vi "Move Drive Encoders.vi"() -> ()   [LabVIEW 2014]
uses:
  Begin/Global RefNums.vi
panel:
  in  "Reset Encoders":bool
  out "BR Current Encoder":i32
  out "BL Current Encoder":i32
  out "FR Current Encoder":i32
  out "FL Current Encoder":i32
  in  "BR Drive Motor":bool
  in  "BL Drive Motor":bool
  in  "FR Drive Motor":bool
  in  "FL Drive Motor":bool
  in  "Drive Back?":bool
  in  "BR Rot Motor":bool
  in  "BL Rot Motor":bool
  in  "FR Rot Motor":bool
  in  "FL Rot Motor":bool
  in  "BR Rot Speed":dbl
  in  "BL Rot Speed":dbl
  in  "FR Rot Speed":dbl
  in  "FL Rot Speed":dbl
  in  "?":bool
  in  "BR Target Encoder":i32
  in  "BL Target Encoder":i32
  in  "FR Target Encoder":i32
  in  "FL Target Encoder":i32
  in  "BR Drive Speed":dbl
  in  "BL Drive Speed":dbl
  in  "FR Drive Speed":dbl
  in  "FL Drive Speed":dbl
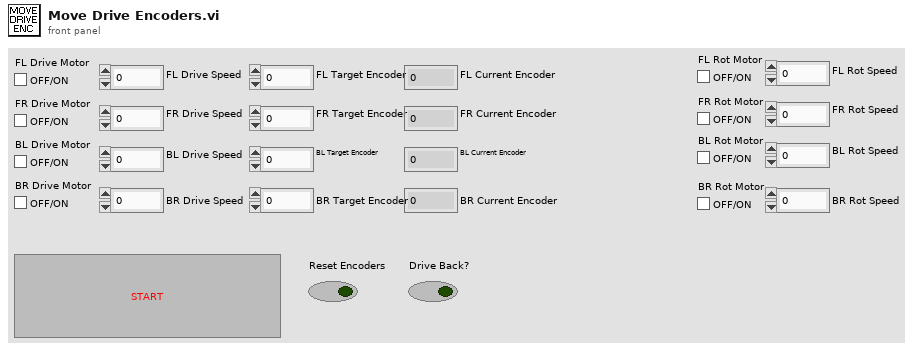
[diagram p1: front panel]
types:
  T1 = typedef "WPI_MotorControlDeviceRef.ctl" = cluster{"DeviceStatus":errorcluster, "Type":T2, "PWM":cluster{"Controller":T3, "PWM Channel":T4, "DeadBand":T5}, "CAN":cluster{"Device Number":u8, "Control Mode":T6, "Semaphore":T7, "Max Vout":dbl, "TalonSRX Control Mode":T8}, "Invert":bool, "TransformRef":T9, "InvTransformRef":T9}
  T2 = typedef "WPI_MotorControlType.ctl" = enum16{"PWM", "CAN", "CANTalonSRX"}
  T3 = typedef "FPGA_TypedefDigitalModule.ctl" = enum16{"Controller 1"}
  T4 = typedef "FPGA_DIOPWMChannel.ctl" = enum8{"PWM 0", "PWM 1", "PWM 2", "PWM 3", "PWM 4", "PWM 5", "PWM 6", "PWM 7", "PWM 8", "PWM 9", "PWM MXP 0", "PWM MXP 1", "PWM MXP 2", "PWM MXP 3", "PWM MXP 4", "PWM MXP 5", "PWM MXP 6", "PWM MXP 7", "PWM MXP 8", "PWM MXP 9", "Invalid"}
  T5 = typedef "WPI_PWMDeadband.ctl" = cluster{"Name":string, "maxPositivePwm":i32, "minPositivePwm":i32, "centerPwm":i32, "maxNegativePwm":i32, "minNegativePwm":i32, "angularRange":u16}
  T6 = typedef "WPI_CANJaguar_ControlMode.ctl" = enum8{"Percent VBus", "Current", "Speed", "Position", "Voltage"}
  T7 = typedef "Semaphore RefNum" = refnum<k1>
  T8 = typedef "WPI_CANTalonSRX_APIControlMode.ctl" = enum8{"Percent VBus", "Speed", "Position", "Slave", "Unchanged / Invalid"}
  T9 = typedef "WPI_PWMTransform_ConPane.ctl" = refnum<vi>
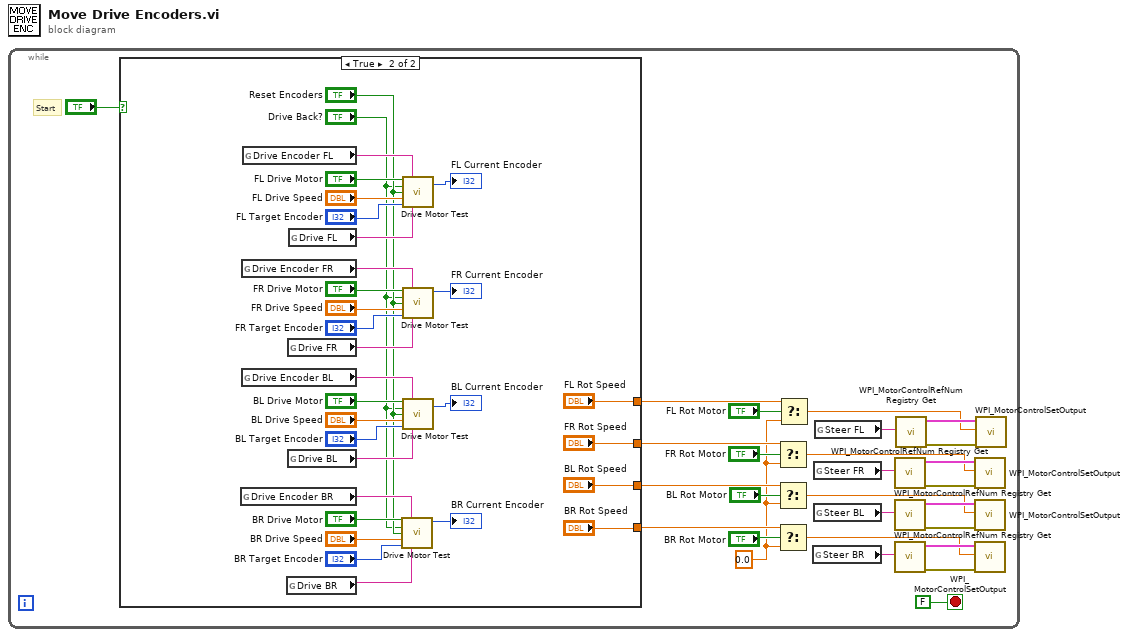
[diagram p0: block diagram]
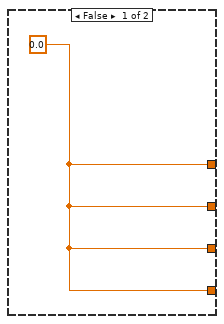
[diagram p2: hidden frame]
diagram:
  n1 = while {
    stop <- FALSE stop-if-true
    w1 = 0.0 ("f")
    # "Start"
    n2 = case shown="True" "?" {
      tunnel: [w28 "FL Rot Speed"] -> w5
      tunnel: [w28 "FR Rot Speed"] -> w4
      tunnel: [w28 "BL Rot Speed"] -> w3
      tunnel: [w28 "BR Rot Speed"] -> w2
      frame False {
        w28 = 0.0 ("FL Drive Speed")
      }
      frame True {
        n3 = global read "Global RefNums.vi" "Drive Encoder BR"() -> (w41:string)
        n4 = global read "Global RefNums.vi" "Drive Encoder FR"() -> (w39:string)
        n5 = global read "Global RefNums.vi" "Drive Encoder BL"() -> (w40:string)
        n6 = global read "Global RefNums.vi" "Drive Encoder FL"() -> (w42:string)
        n7 = global read "Global RefNums.vi" "Drive BR"() -> (w35:string)
        n8 = global read "Global RefNums.vi" "Drive FR"() -> (w37:string)
        n9 = global read "Global RefNums.vi" "Drive BL"() -> (w36:string)
        n10 = global read "Global RefNums.vi" "Drive FL"() -> (w38:string)
        n11 = call "Drive Motor Test.vi"("On?"="BR Drive Motor", "Encoder Refnum"=w41, "Drive Back?"="Drive Back?", "Reset Encoders"="Reset Encoders", "Speed"="BR Drive Speed", "Target Encoder"="BR Target Encoder", "Motor Refnum"=w35) -> ("Current Encoder"=→"BR Current Encoder":i32)  [unwired: 8 in]
        n12 = call "Drive Motor Test.vi"("On?"="FL Drive Motor", "Encoder Refnum"=w42, "Drive Back?"="Drive Back?", "Reset Encoders"="Reset Encoders", "Speed"="FL Drive Speed", "Target Encoder"="FL Target Encoder", "Motor Refnum"=w38) -> ("Current Encoder"=→"FL Current Encoder":i32)  [unwired: 8 in]
        n13 = call "Drive Motor Test.vi"("On?"="FR Drive Motor", "Encoder Refnum"=w39, "Drive Back?"="Drive Back?", "Reset Encoders"="Reset Encoders", "Speed"="FR Drive Speed", "Target Encoder"="FR Target Encoder", "Motor Refnum"=w37) -> ("Current Encoder"=→"FR Current Encoder":i32)  [unwired: 8 in]
        n14 = call "Drive Motor Test.vi"("On?"="BL Drive Motor", "Encoder Refnum"=w40, "Drive Back?"="Drive Back?", "Reset Encoders"="Reset Encoders", "Speed"="BL Drive Speed", "Target Encoder"="BL Target Encoder", "Motor Refnum"=w36) -> ("Current Encoder"=→"BL Current Encoder":i32)  [unwired: 8 in]
      }
    }
    n15 = Select(t=w4, s="FR Rot Motor", f=w1) -> (s? t:f=w12:dbl)
    n16 = Select(t=w3, s="BL Rot Motor", f=w1) -> (s? t:f=w11:dbl)
    n17 = Select(t=w2, s="BR Rot Motor", f=w1) -> (s? t:f=w10:dbl)
    n18 = Select(t=w5, s="FL Rot Motor", f=w1) -> (s? t:f=w13:dbl)
    n19 = global read "Global RefNums.vi" "Steer BR"() -> (w17:string)
    n20 = global read "Global RefNums.vi" "Steer FR"() -> (w23:string)
    n21 = global read "Global RefNums.vi" "Steer BL"() -> (w20:string)
    n22 = global read "Global RefNums.vi" "Steer FL"() -> (w14:string)
    n23 = call <vilib>:"WPI_MotorControlRefNum Registry Get.vi"("refnum name"=w23) -> ("error out"=w24:errorcluster, "MotorControlDevRef"=w25:T1)  [unwired: 9 in]
    n24 = call <vilib>:"WPI_MotorControlRefNum Registry Get.vi"("refnum name"=w20) -> ("error out"=w21:errorcluster, "MotorControlDevRef"=w22:T1)  [unwired: 9 in]
    n25 = call <vilib>:"WPI_MotorControlRefNum Registry Get.vi"("refnum name"=w17) -> ("error out"=w18:errorcluster, "MotorControlDevRef"=w19:T1)  [unwired: 9 in]
    n26 = call <vilib>:"WPI_MotorControlRefNum Registry Get.vi"("refnum name"=w14) -> ("error out"=w15:errorcluster, "MotorControlDevRef"=w16:T1)  [unwired: 9 in]
    n27 = call <vilib>:"WPI_MotorControlSetOutput.vi"("error in (no error)"=w24, "Output"=w12, "MotorControlDevRef"=w25) -> ()  [unwired: 6 in, 3 out]
    n28 = call <vilib>:"WPI_MotorControlSetOutput.vi"("error in (no error)"=w21, "Output"=w11, "MotorControlDevRef"=w22) -> ()  [unwired: 6 in, 3 out]
    n29 = call <vilib>:"WPI_MotorControlSetOutput.vi"("error in (no error)"=w18, "Output"=w10, "MotorControlDevRef"=w19) -> ()  [unwired: 6 in, 3 out]
    n30 = call <vilib>:"WPI_MotorControlSetOutput.vi"("error in (no error)"=w15, "Output"=w13, "MotorControlDevRef"=w16) -> ()  [unwired: 6 in, 3 out]
  }
